vi "ex3.vi"() -> ()   [LabVIEW 2017]
uses:
  <vilib>/sound2/lvsound2.llb/Sound File Read Open.vi
  <vilib>/sound2/lvsound2.llb/Sound File Info (refnum).vi
  <vilib>/sound2/lvsound2.llb/Sound File Read (DBL).vi
panel:
  out "Waveform Chart":waveform(dbl)[](graph)
  in  "path":path
  in  "stop":bool
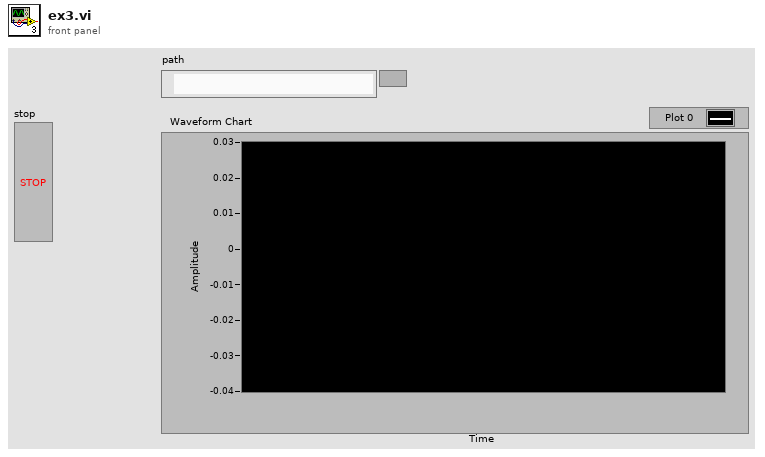
[diagram p1: front panel]
types:
  T1 = typedef "Sound File Refnum.ctl" = refnum<file>
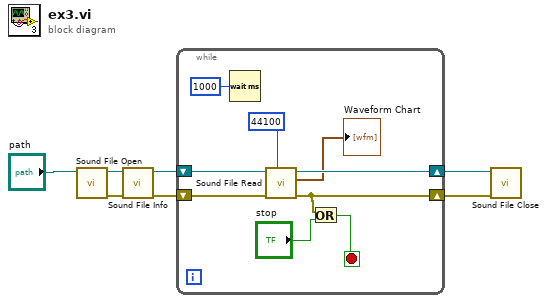
[diagram p0: block diagram]
diagram:
  n1 = call-poly <vilib>:"Sound File Open.vi"("path"="path") -> ("error out"=w7:errorcluster, "sound file refnum"=w4:T1)  [unwired: 9 in]
  n2 = call-poly <vilib>:"Sound File Info.vi"("error in (no error)"=w7, "sound file refnum"=w4) -> ("error out"=w6:errorcluster, "sound file refnum out"=w3:T1)  [unwired: 6 in, 2 out]
  n3 = while {
    shift-right: [w13] -> w5
    shift-left: w6 -> [w16]
    shift-right: [w14] -> w2
    shift-left: w3 -> [w15]
    stop <- w11 stop-if-true
    n4 = Wait (ms)(milliseconds to wait=u32 1000) -> ()  [unwired: 1 out]
    n5 = call-poly <vilib>:"Sound File Read.vi"("number of samples/ch (-1: all)"=44100, "error in (no error)"=w16, "sound file refnum"=w15) -> ("error out"=w13:errorcluster, "data"=→"Waveform Chart":waveform(dbl)[], "sound file refnum out"=w14:T1)  [unwired: 4 in, 2 out]
    n6 = Or(x=w13, y="stop") -> (x .or. y?=w11:bool)
  }
  n7 = call <vilib>:"Sound File Close.vi"("error in (no error)"=w5, "sound file refnum"=w2) -> ()  [unwired: 9 in, 1 out]
